vi "finduntracComport.vi"() -> (8 "OUT COM":refnum<visa-resource-name>, 10 "error out":errorcluster)   [LabVIEW 2014]
uses:
  <vilib>/Instr/_visa.llb/VISA Find Search Mode.ctl
  <vilib>/Instr/_visa.llb/VISA Configure Serial Port (Instr).vi
panel:
  out "find list":string[](array[string])
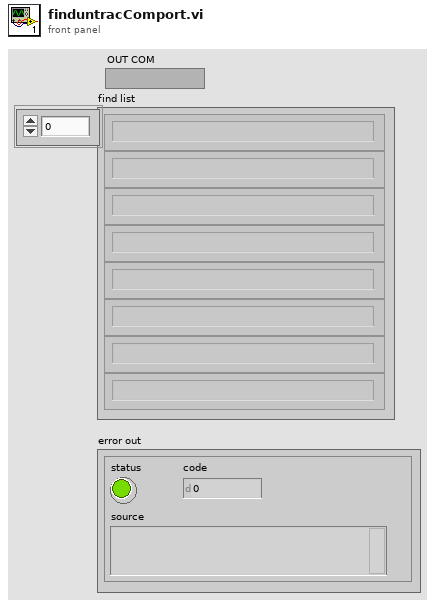
[diagram p1: front panel]
types:
  T1 = typedef "VISA Find Search Mode.ctl" = u32
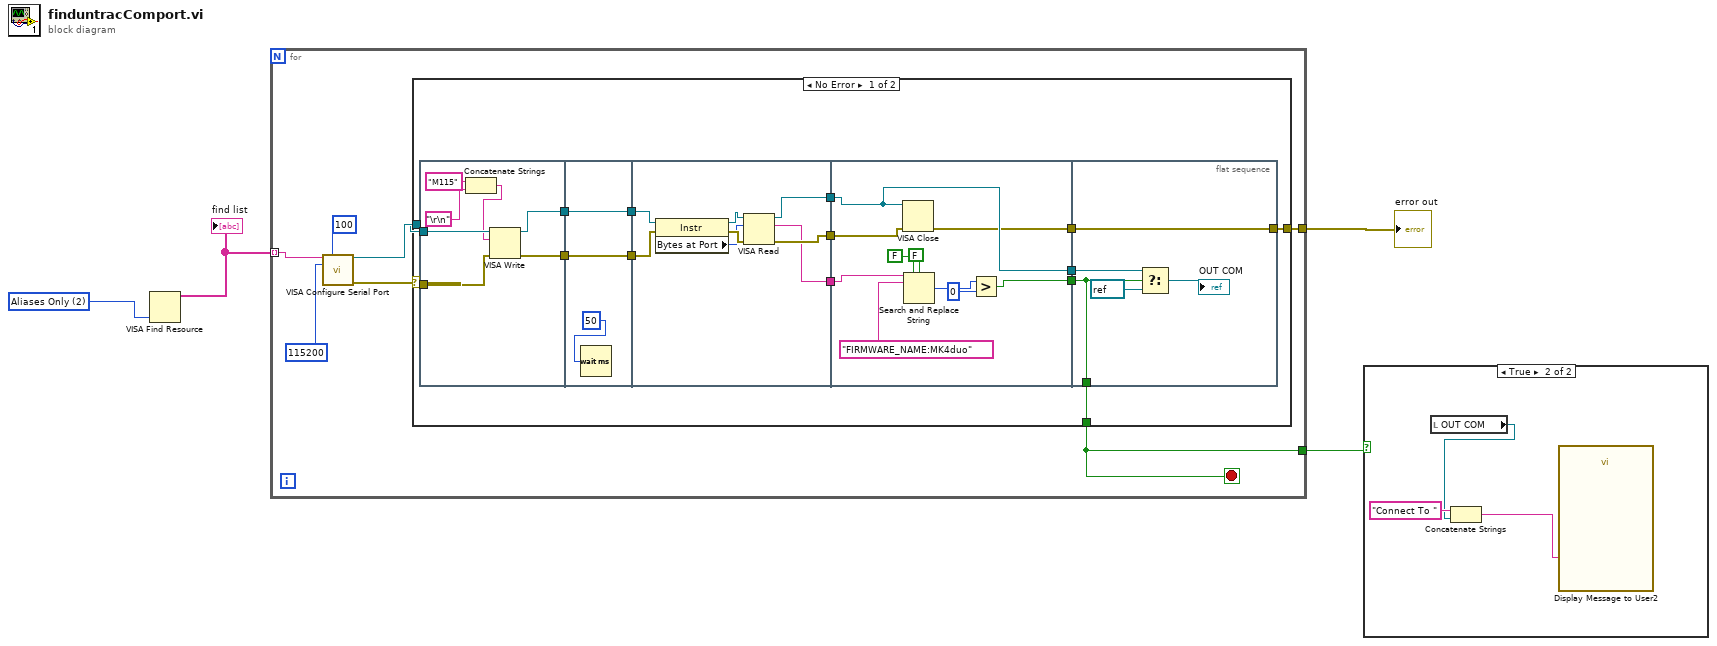
[diagram p0: block diagram]
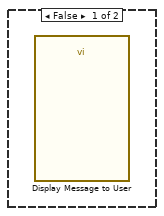
[diagram p2: hidden frame]
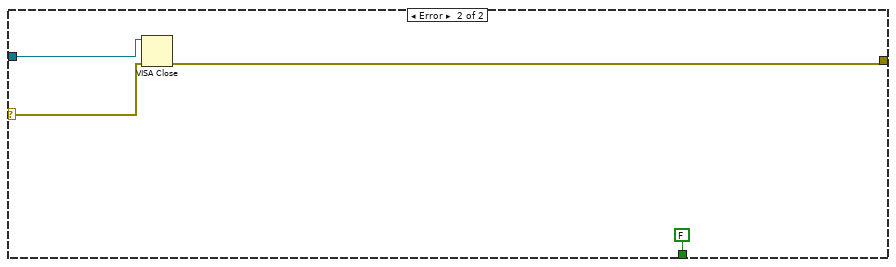
[diagram p3: hidden frame]
diagram:
  w4 = T1 2 items=["Canonical Names Only"=0, "Aliases Only"=2, "Include Matching Aliases"=3, "Include All Aliases"=4] ("Search Mode")
  n1 = VISA Find Resource(10:w4) -> (3:w3:string[])  [unwired: 2 in, 2 out]
  "find list" <- w3
  n2 = for {
    tunnel: w3 -> [w6] mode=indexing
    tunnel: [w8] -> w2
    tunnel: [w5] -> w1
    stop <- w5 stop-if-true
    n3 = call-poly "VISA Configure Serial Port"("VISA resource name"=w6, "timeout (10sec)"=u32 100, "baud rate (9600)"=u32 115200) -> ("VISA resource name out"=w10:refnum<visa-resource-name>, "error out"=w11:errorcluster)  [unwired: 11 in]
    n4 = case shown="No Error" w11 {
      selector: w11 -> [w20 w61]
      tunnel: w10 -> [w21 w62]
      tunnel: [w13 w60] -> w8
      tunnel: [w12 FALSE] -> w5
      frame No Error {
        n5 = flat-sequence {
          tunnel: [w31] -> w25
          tunnel: [w30] -> w24
          tunnel: w21 -> [w32]
          tunnel: w20 -> [w27]
          tunnel: [w34] -> w23
          tunnel: w25 -> [w34]
          tunnel: w24 -> [w33]
          tunnel: [w33] -> w22
          tunnel: w23 -> [w41]
          tunnel: w22 -> [w40]
          tunnel: [w43] -> w19
          tunnel: [w42] -> w18
          tunnel: [w36] -> w17
          tunnel: w19 -> [w50]
          tunnel: w18 -> [w49]
          tunnel: w17 -> [w45]
          tunnel: [w46] -> w16
          tunnel: [w45] -> w15
          tunnel: [w44] -> w14
          tunnel: w16 -> [w54]
          tunnel: w15 -> [w58]
          tunnel: [w56] -> w13
          tunnel: w14 -> [w56]
          tunnel: [w54] -> w12
          frame #0 {
            n6 = Concatenate Strings("M115" ("string"), "\r\n") -> (w28:string)
            n7 = VISA Write(VISA resource name=w32, write buffer=w28, error in (no error)=w27) -> (VISA resource name out=w31:refnum<visa-resource-name>, error out=w30:errorcluster)  [unwired: 1 out]
          }
          frame #1 {
            n8 = Wait (ms)(milliseconds to wait=u32 50 ("millisecond timer value")) -> ()  [unwired: 1 out]
          }
          frame #2 {
            n9 = property class="Instr"(reference=w41, error in=w40) -> (reference out=w39:refnum<visa-resource-name>, error out=w38:errorcluster, "Bytes at Port"=w37:u32)
            n10 = VISA Read(VISA resource name=w39, byte count=w37, error in (no error)=w38) -> (VISA resource name out=w36:refnum<visa-resource-name>, read buffer=w42:string, error out=w43:errorcluster)  [unwired: 1 out]
          }
          frame #3 {
            n11 = VISA Close(VISA resource name=w45, error in (no error)=w50) -> (error out=w44:errorcluster)
            n12 = Search and Replace String(replace all?=FALSE ("replace all? (F)"), case sensitive?=FALSE ("ignore case? (F)"), input string=w49, search string="FIRMWARE_NAME:MK4duo") -> (number of replacements=w48:i32)  [unwired: 4 in, 3 out]
            n13 = Greater?(x=w48, y=0) -> (0:w46:bool)
          }
          frame #4 {
            n14 = Select(t=w58, s=w54, f=refnum<visa-resource-name> refnum) -> (s? t:f=→"OUT COM":refnum<visa-resource-name>)
          }
        }
      }
      frame Error {
        n15 = VISA Close(VISA resource name=w62, error in (no error)=w61) -> (error out=w60:errorcluster)
      }
    }
  }
  "error out" <- w2
  n16 = case shown="True" w1 {
    frame False {
      n17 = call "Display Message to User"() -> ()  [unwired: 10 in, 2 out]
    }
    frame True {
      n18 = local read "OUT COM"() -> (w63:refnum<visa-resource-name>)
      n19 = Concatenate Strings("Connect To " ("string"), w63) -> (w65:string)
      n20 = call "Display Message to User2"("Message"=w65) -> ()  [unwired: 9 in, 2 out]
    }
  }
